vi "UART_StopExternalSupply.vi"(7 "Setling (s)":dbl, 8 "error in (no error)":errorcluster, 10 "pin":string, 11 "IVI Refnum in":refnum<k15>) -> (0 "error out":errorcluster, 3 "IVI Refnum out":refnum<k15>)   [LabVIEW 2024, in "UART.lvlib"]
doc: "Set the external supply to 0V and wait the amount of Settling (s)"
uses:
  UART.lvlib
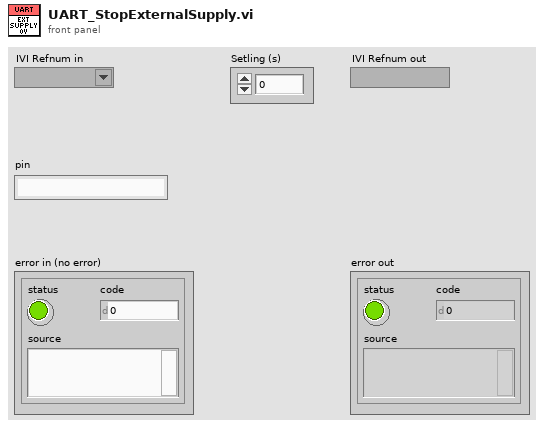
[diagram p1: front panel]
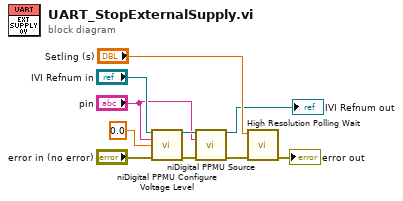
[diagram p0: block diagram]
diagram:
  n1 = call <instrlib>:"niDigital PPMU Configure Voltage Level.vi"("instrument handle"="IVI Refnum in", "channel list"="pin", "voltage level (V)"=0.0, "error in"="error in (no error)") -> ("instrument handle out"=w6:refnum<k15>, "error out"=w5:errorcluster)  [unwired: 10 in]
  n2 = call <instrlib>:"niDigital PPMU Source.vi"("instrument handle"=w6, "channel list"="pin", "error in"=w5) -> ("instrument handle out"=→"IVI Refnum out":refnum<k15>, "error out"=w8:errorcluster)  [unwired: 11 in]
  n3 = call <vilib>:"High Resolution Polling Wait.vi"("error in (no error)"=w8, "seconds to wait"="Setling (s)") -> ("error out"=→"error out":errorcluster)  [unwired: 9 in]
